vi "Open_his_files.vi"(8 "error in (no error)":errorcluster, 11 "dict of HIS IN":variant) -> (0 "error out":errorcluster, 3 "dict of HIS OUT":variant)   [LabVIEW 2015]
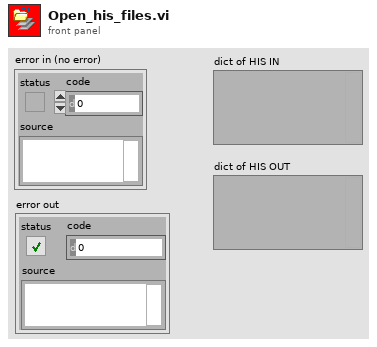
[diagram p1: front panel]
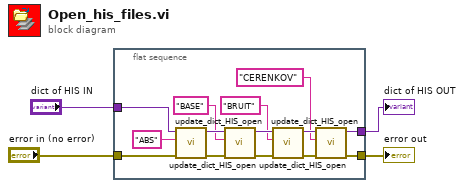
[diagram p0: block diagram]
diagram:
  n1 = flat-sequence {
    tunnel: "dict of HIS IN" -> [w18]
    tunnel: [w14] -> w3
    tunnel: "error in (no error)" -> [w13]
    tunnel: [w9] -> w1
    frame #0 {
      n2 = call "update_dict_HIS_open.vi"("error in (no error)"=w13, "type"="ABS" ("name"), "dict of HIS IN"=w18) -> ("error out"=w12:errorcluster, "dict of HIS OUT"=w17:variant)  [unwired: 7 in]
      n3 = call "update_dict_HIS_open.vi"("error in (no error)"=w12, "type"="BASE" ("name"), "dict of HIS IN"=w17) -> ("error out"=w11:errorcluster, "dict of HIS OUT"=w16:variant)  [unwired: 7 in]
      n4 = call "update_dict_HIS_open.vi"("error in (no error)"=w11, "type"="BRUIT" ("name"), "dict of HIS IN"=w16) -> ("error out"=w10:errorcluster, "dict of HIS OUT"=w15:variant)  [unwired: 7 in]
      n5 = call "update_dict_HIS_open.vi"("error in (no error)"=w10, "type"="CERENKOV" ("name"), "dict of HIS IN"=w15) -> ("error out"=w9:errorcluster, "dict of HIS OUT"=w14:variant)  [unwired: 7 in]
    }
  }
  "dict of HIS OUT" <- w3
  "error out" <- w1
